vi "Add.vi"(8 "error in":errorcluster, 9 "configuration version":cluster{"major":u32, "minor":u32, "fix":u32}={"major"=1, "minor"=0, "fix"=0}, 10 "framework configuration":T1, 11 "target in":refnum<k24>) -> (0 "error out":errorcluster, 2 "data sharing framework custom device":T17 format="%.0x", 3 "target out":refnum<k24>)   [LabVIEW 2020, in "Data Sharing Framework Custom Device Scripting.lvlib"]
doc: "For the <b>specified target in</b>, adds a new instance of the Data Sharing Framework custom device to the system definition."
uses:
  Data Sharing Framework Custom Device Scripting.lvlib
  NationalInstruments.VeriStand.SystemDefinitionAPI
  <vilib>/NI VeriStand/Custom Device API/Custom Device Item Ref.ctl
  Includes/DSF Core.lvlibp/Typedefs/DSF Engine Framework Configuration.ctl
  Includes/DSF Core.lvlibp/Typedefs/DSF Engine Plugin Configuration.ctl
  Includes/DSF Core.lvlibp/Typedefs/Core Plugin Configuration.ctl
  Includes/DSF Core.lvlibp/Typedefs/DSF Timing Info.ctl
  Includes/DSF Core.lvlibp/Typedefs/DSF Settings Info.ctl
  Includes/DSF Core.lvlibp/Typedefs/DSF Engine Plugin Thread Configuration.ctl
  Includes/DSF Core.lvlibp/Typedefs/Core Thread Configuration.ctl
  Includes/DSF Core.lvlibp/Typedefs/DSF Engine Transfer Group Configuration.ctl
  Includes/DSF Core.lvlibp/Typedefs/Core Group Configuration.ctl
  Includes/DSF Core.lvlibp/Typedefs/DSF Direction.ctl
  Includes/DSF Core.lvlibp/Typedefs/DSF Timeout Behavior.ctl
  Includes/DSF Core.lvlibp/Typedefs/DSF Engine Transfer Configuration.ctl
  Includes/DSF Core.lvlibp/Typedefs/Core Transfer Configuration.ctl
  Includes/DSF Core.lvlibp/Typedefs/DSF Engine Channel Configuration.ctl
  Includes/DSF Core.lvlibp/Typedefs/Core Channel Configuration.ctl
  Includes/DSF Core.lvlibp/Typedefs/DSF Data Type.ctl
  Shared/DSF Shared.lvlib
  System Explorer/DSF System Explorer.lvlib
  <vilib>/NI VeriStand/Custom Device API/Custom Device API.lvlib
  Includes/DSF Core.lvlibp
  Includes/DSF Core.lvlibp/Classes/Configuration/Core/Plugin/Plugin Configuration.lvclass
  Includes/DSF Core.lvlibp/Classes/Configuration/Core/Thread/Thread Configuration.lvclass
  Includes/DSF Core.lvlibp/Classes/Configuration/Core/Group/Group Configuration.lvclass
  Includes/DSF Core.lvlibp/Classes/Configuration/Core/Transfer/Transfer Configuration.lvclass
  Includes/DSF Core.lvlibp/Classes/Configuration/Core/Channel/Channel Configuration.lvclass
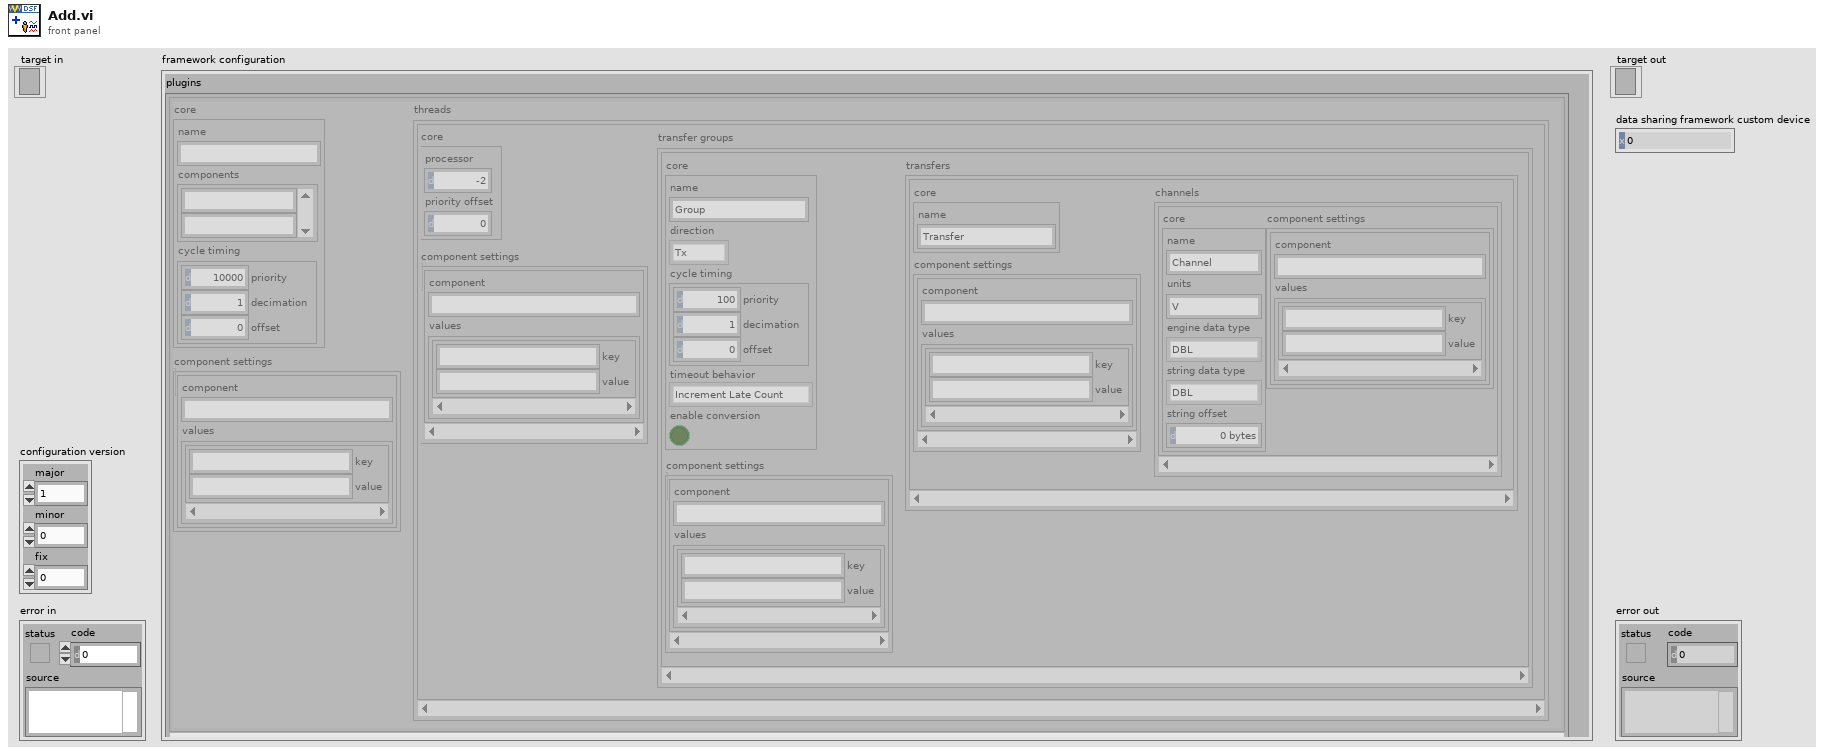
[diagram p1: front panel]
types:
  T1 = typedef "DSF Core.lvlibp/DSF Engine Framework Configuration.ctl" = cluster{"plugins":T2[]}
  T2 = typedef "DSF Core.lvlibp/DSF Engine Plugin Configuration.ctl" = cluster{"core":T3, "component settings":T5[], "threads":T6[]}
  T3 = typedef "DSF Core.lvlibp/Plugin Configuration.lvclass/Core Plugin Configuration.ctl" = cluster{"name":string, "components":string[], "cycle timing":T4}
  T4 = typedef "DSF Core.lvlibp/DSF Timing Info.ctl" = cluster{"priority":u64, "decimation":u64, "offset":u64}
  T5 = typedef "DSF Core.lvlibp/DSF Settings Info.ctl" = cluster{"component":string, "values":cluster{"key":string, "value":string}[]}
  T6 = typedef "DSF Core.lvlibp/DSF Engine Plugin Thread Configuration.ctl" = cluster{"core":T7, "component settings":T5[], "transfer groups":T8[]}
  T7 = typedef "DSF Core.lvlibp/Thread Configuration.lvclass/Core Thread Configuration.ctl" = cluster{"processor":i32, "priority offset":i16}
  T8 = typedef "DSF Core.lvlibp/DSF Engine Transfer Group Configuration.ctl" = cluster{"core":T9, "component settings":T5[], "transfers":T12[]}
  T9 = typedef "DSF Core.lvlibp/Group Configuration.lvclass/Core Group Configuration.ctl" = cluster{"name":string, "direction":T10, "cycle timing":T4, "timeout behavior":T11, "enable conversion":bool}
  T10 = typedef "DSF Core.lvlibp/DSF Direction.ctl" = enum8{"Tx", "Rx"}
  T11 = typedef "DSF Core.lvlibp/DSF Timeout Behavior.ctl" = enum8{"Increment Late Count", "Throw Error"}
  T12 = typedef "DSF Core.lvlibp/DSF Engine Transfer Configuration.ctl" = cluster{"core":T13, "component settings":T5[], "channels":T14[]}
  T13 = typedef "DSF Core.lvlibp/Transfer Configuration.lvclass/Core Transfer Configuration.ctl" = cluster{"name":string}
  T14 = typedef "DSF Core.lvlibp/DSF Engine Channel Configuration.ctl" = cluster{"core":T15, "component settings":T5[]}
  T15 = typedef "DSF Core.lvlibp/Channel Configuration.lvclass/Core Channel Configuration.ctl" = cluster{"name":string, "units":string, "engine data type":T16, "string data type":T16, "string offset":u64}
  T16 = typedef "DSF Core.lvlibp/DSF Data Type.ctl" = enum8{"Bool", "SGL", "DBL", "I8", "I16", "I32", "I64", "U8", "U16", "U32", "U64"}
  T17 = typedef "Custom Device API.lvlib/Custom Device Item Ref.ctl" = u64
  T18 = typedef "DSF Core.lvlibp/DSF Version Info.ctl" = cluster{"major":u32, "minor":u32, "fix":u32, "build":string}
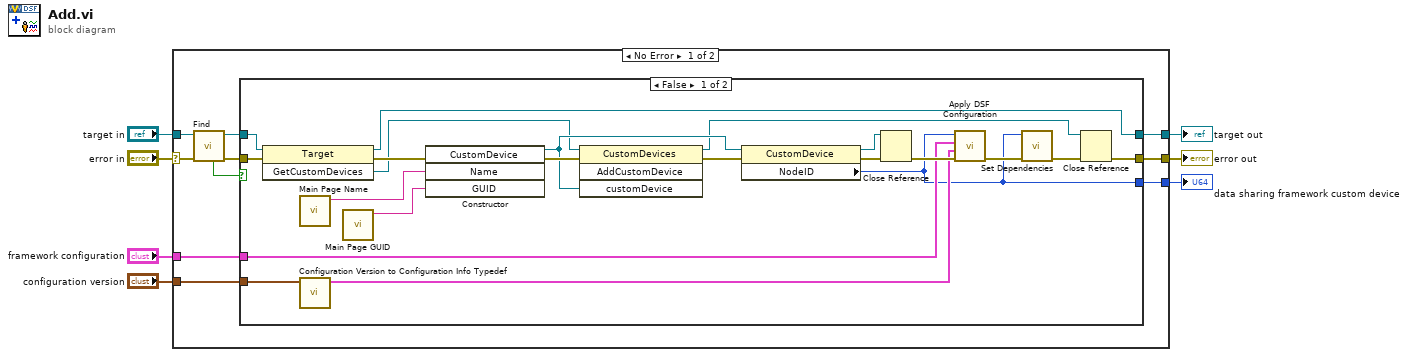
[diagram p0: block diagram]
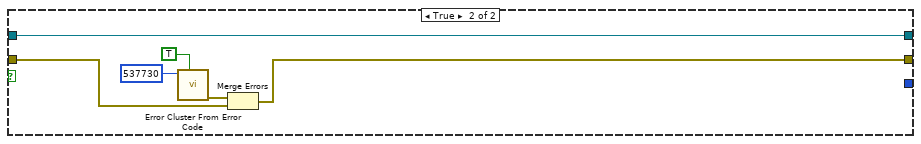
[diagram p2: hidden frame]
diagram:
  n1 = case shown="No Error" "error in" {
    selector: "error in" -> [w15 w46]
    tunnel: [w11 w46] -> w7
    tunnel: "target in" -> [w16 w45]
    tunnel: [w12 w45] -> w4
    tunnel: [w17 _] -> w3
    tunnel: "framework configuration" -> [w10 _]
    tunnel: "configuration version" -> [w9 _]
    frame No Error {
      n2 = call "Find.vi"("error in"=w15, "target in"=w16) -> ("error out"=w13:errorcluster, "target out"=w14:refnum<k24>, "found?"=w8:bool)  [unwired: 6 in, 1 out]
      n3 = case shown="False" w8 {
        tunnel: [w25 w42] -> w11
        tunnel: [w18 _] -> w17
        tunnel: w14 -> [w31 w40]
        tunnel: w13 -> [w30 w41]
        tunnel: [w29 w40] -> w12
        tunnel: w10 -> [w22 _]
        tunnel: w9 -> [w21 _]
        frame False {
          n4 = invoke class="Target" method="GetCustomDevices"(reference=w31, error in=w30) -> (reference out=w29:refnum<k24>, error out=w28:errorcluster, "GetCustomDevices"=w27:refnum<k24>)  [unwired: 1 in]
          n5 = call "Main Page Name.vi"() -> ("name"=w34:string)  [unwired: 11 in]
          n6 = call "Configuration Version to Configuration Info Typedef.vi"("configuration version"=w21) -> ("version info"=w20:T18)  [unwired: 10 in]
          n7 = call "Main Page GUID.vi"() -> ("Main Page GUID"=w32:string)  [unwired: 11 in]
          n8 = constructor class="CustomDevice"(error in=w28, "Name"=w34, "GUID"=w32) -> (reference out=w33:refnum<k24>, error out=w38:errorcluster)  [unwired: 2 in, 3 out]
          n9 = invoke class="CustomDevices" method="AddCustomDevice"(reference=w27, error in=w38, "customDevice"=w33) -> (reference out=w26:refnum<k24>, error out=w37:errorcluster)  [unwired: 1 in, 2 out]
          n10 = property class="CustomDevice"(reference=w33, error in=w37) -> (reference out=w36:refnum<k24>, error out=w35:errorcluster, "NodeID"=w18:u64)
          n11 = Close Reference(reference=w36, error in (no error)=w35) -> (error out=w24:errorcluster)
          n12 = call "Apply DSF Configuration.vi"("error in (no error)"=w24, "version"=w20, "framework configuration"=w22, "Item Ref in"=w18) -> ("error out"=w23:errorcluster)  [unwired: 7 in]
          n13 = call "Set Dependencies.vi"("error in (no error)"=w23, "Device Item Ref in"=w18) -> ("error out"=w19:errorcluster)  [unwired: 8 in, 1 out]
          n14 = Close Reference(reference=w26, error in (no error)=w19) -> (error out=w25:errorcluster)
        }
        frame True {
          n15 = call <vilib>:"Error Cluster From Error Code.vi"("show call chain? (False)"=TRUE, "error code (0)"=537730) -> ("error out"=w43:errorcluster)  [unwired: 7 in]
          n16 = Merge Errors(w43, w41) -> (w42:errorcluster)
        }
      }
    }
    frame Error {
    }
  }
  "target out" <- w4
  "error out" <- w7
  "data sharing framework custom device" <- w3
